vi "Display Data Queue 32bit.vi"(4 "timeout in ms (-1)":i32=10, 6 "max queue size (-1, unlimited)":i32, 7 "Action":T1=enum."Enqueue", 8 "error in (no error)":errorcluster, 11 "data in":sgl[](array[numeric])) -> (0 "error out":errorcluster, 1 "Empty?":bool, 2 "# elements in queue":i32, 3 "data out":sgl[](array[numeric]))   [LabVIEW 2018]
uses:
  Controls/Queue Manager Actions.ctl
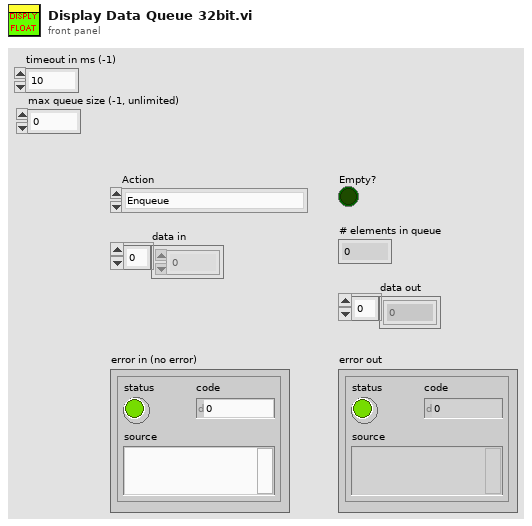
[diagram p1: front panel]
types:
  T1 = typedef "Queue Manager Actions.ctl" = enum16{"Init", "Enqueue", "Enqueue All", "Preview Queue", "Dequeue", "Get Status", "Flush Queue", "Flush All Queues", "Release All Queues", "Release Queue", "Enqueue at Opposite End"}
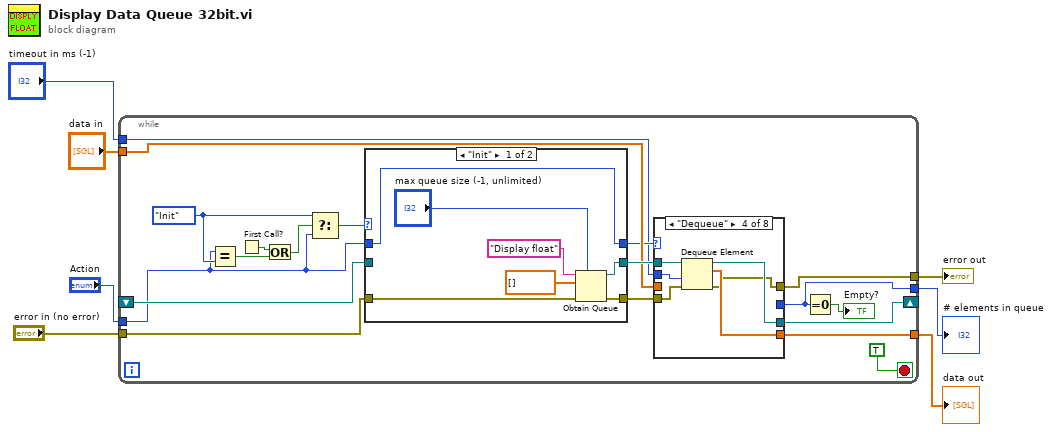
[diagram p0: block diagram]
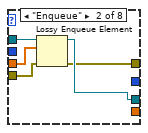
[diagram p3: hidden frame]
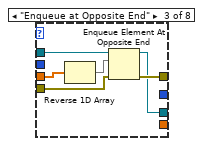
[diagram p4: hidden frame]
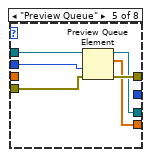
[diagram p5: hidden frame]
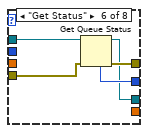
[diagram p6: hidden frame]
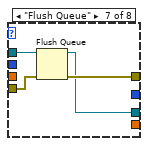
[diagram p7: hidden frame]
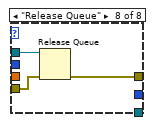
[diagram p8: hidden frame]
diagram:
  n1 = while {
    tunnel: "Action" -> [w9]
    tunnel: "error in (no error)" -> [w14]
    shift-right: [w16] -> _
    shift-left: _ -> [w15]
    tunnel: "data in" -> [w12]
    tunnel: "timeout in ms (-1)" -> [w8]
    tunnel: [w19] -> w3
    tunnel: [w18] -> w2
    tunnel: [w11] -> w1
    stop <- TRUE stop-if-true
    w21 = Queue_Manager_Actions."Init"
    n2 = Equal?(x=w9, y=w21) -> (x = y?=w23:bool)
    n3 = First Call?() -> (First Call?: T/F=w24:bool)
    n4 = Or(x=w24, y=w23) -> (x .or. y?=w22:bool)
    n5 = Select(t=w21, s=w22, f=w9) -> (s? t:f=w20:T1)
    n6 = case shown="\"Init\"" w20 {
      tunnel: [w70 w73] -> w17
      tunnel: [w69 w72] -> w13
      tunnel: w15 -> [_ w73]
      tunnel: w14 -> [w67 w72]
      tunnel: [w65 w71] -> w10
      tunnel: w9 -> [w65 w71]
      frame "Init" {
        n7 = Obtain Queue(max queue size (-1, unlimited)="max queue size (-1, unlimited)", name (unnamed)="Display float", element data type=sgl[] [], error in (no error)=w67) -> (queue out=w70:refnum<queue>, error out=w69:errorcluster)  [unwired: 1 in, 1 out]
      }
      frame Default {
      }
    }
    n8 = case shown="\"Dequeue\"" w10 {
      tunnel: [w27 w29 w39 w40 w51 w56 w60 w63] -> w19
      tunnel: [_ _ _ w45 w50 _ _ _] -> w18
      tunnel: [_ _ _ _ _ w55 _ _] -> w11
      tunnel: w17 -> [w28 w33 w36 w44 w48 w54 w59 w62]
      tunnel: [w28 w30 w37 w41 w47 w52 w57 _] -> w16
      tunnel: w13 -> [w27 w32 w35 w43 w49 w53 w58 w61]
      tunnel: w12 -> [_ w31 w34 _ _ _ _ _]
      tunnel: w8 -> [_ _ _ w42 w46 _ _ _]
      frame "Init", Default {
      }
      frame "Enqueue" {
        n9 = Lossy Enqueue Element(queue=w33, element=w31, error in (no error)=w32) -> (queue out=w30:refnum<queue>, error out=w29:errorcluster)  [unwired: 2 out]
      }
      frame "Enqueue at Opposite End" {
        n10 = Reverse 1D Array(array=w34) -> (reversed array=w38:sgl[])
        n11 = Enqueue Element At Opposite End(queue=w36, element=w38, error in (no error)=w35) -> (queue out=w37:refnum<queue>, error out=w39:errorcluster)  [unwired: 1 in, 1 out]
      }
      frame "Dequeue" {
        n12 = Dequeue Element(queue=w44, timeout in ms (-1)=w42, error in (no error)=w43) -> (queue out=w41:refnum<queue>, element=w45:sgl[], error out=w40:errorcluster)  [unwired: 1 out]
      }
      frame "Preview Queue" {
        n13 = Preview Queue Element(queue=w48, timeout in ms (-1)=w46, error in (no error)=w49) -> (queue out=w47:refnum<queue>, element=w50:sgl[], error out=w51:errorcluster)  [unwired: 1 out]
      }
      frame "Get Status" {
        n14 = Get Queue Status(queue=w54, error in (no error)=w53) -> (queue out=w52:refnum<queue>, error out=w56:errorcluster, # elements in queue=w55:i32)  [unwired: 1 in, 5 out]
      }
      frame "Flush Queue" {
        n15 = Flush Queue(queue=w59, error in (no error)=w58) -> (queue out=w57:refnum<queue>, error out=w60:errorcluster)  [unwired: 1 out]
      }
      frame "Release Queue" {
        n16 = Release Queue(queue=w62, error in (no error)=w61) -> (error out=w63:errorcluster)  [unwired: 1 in, 2 out]
      }
    }
    n17 = Equal To 0?(x=w11) -> (x = 0?=→"Empty?":bool)
  }
  "error out" <- w3
  "data out" <- w2
  "# elements in queue" <- w1
